vi "mqttTCPIPbrokerConnect.vi"(0 "mqtt in":refnum<class "mqtt.lvclass">, 11 "error in (no error)":errorcluster) -> (4 "mqtt out":refnum<class "mqtt.lvclass">, 15 "error out":errorcluster)   [LabVIEW 2018, in "mqtt.lvclass"]
uses:
  mqtt.lvclass
  mqtt.lvclass/mqtt.ctl
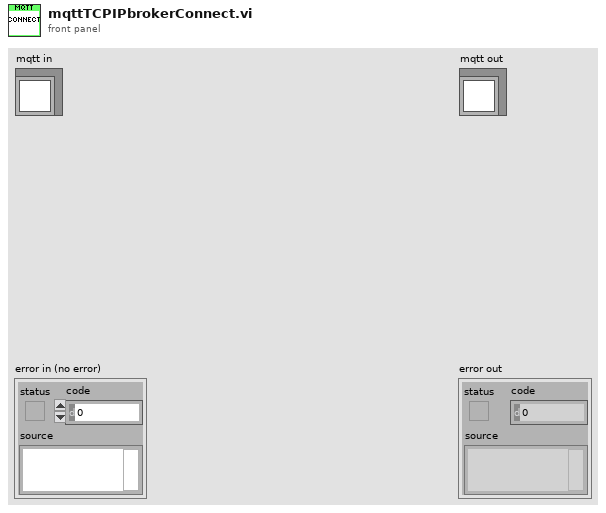
[diagram p1: front panel]
types:
  T1 = typedef "mqttBroker.ctl" = cluster{"address":string, "port":u16, "connTimeout":i32, "writeTimeout":i32, "readTimeout":i32, "subTimeout":i32}
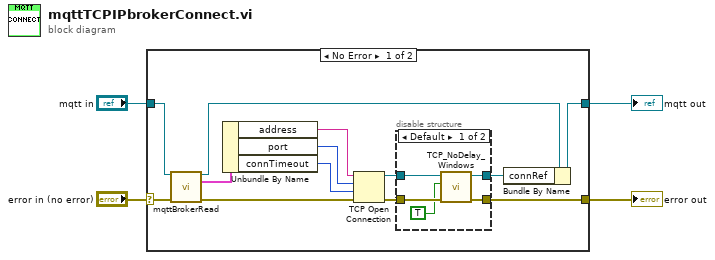
[diagram p0: block diagram]
diagram:
  n1 = case shown="No Error" "error in (no error)" {
    selector: "error in (no error)" -> [w14 w26]
    tunnel: [w15 w26] -> w3
    tunnel: [w5 w25] -> w1
    tunnel: "mqtt in" -> [w9 w25]
    frame No Error {
      n2 = call "mqttBrokerRead.vi"("mqtt in"=w9, "error in (no error)"=w14) -> ("mqtt out"=w7:refnum<class "mqtt.lvclass">, "broker"=w12:T1, "error out"=w13:errorcluster)  [unwired: 11 in]
      n3 = Unbundle By Name(w12) -> ("address"=w11:string, "port"=w10:u16, "connTimeout"=w8:i32)
      n4 = TCP Open Connection(address=w11, remote port or service name=w10, timeout ms (60000)=w8, error in (no error)=w13) -> (connection ID=w17:refnum<k5>, error out=w16:errorcluster)  [unwired: 1 in]
      n5 = disable-structure shown="Default" {
        disable-tunnel: w17 -> [w22 w24]
        disable-tunnel: w16 -> [w21 w23]
        disable-tunnel: [w20 w23] -> w15
        disable-tunnel: [w18 w24] -> w6
        frame condition #0 (active) {
          n6 = call "TCP_NoDelay_Windows.vi"("error in (no error)"=w21, "TCP_NODELAY (true)"=TRUE, "connID"=w22) -> ("error out"=w20:errorcluster, "connID 2"=w18:refnum<k5>)  [unwired: 3 in]
        }
        frame condition #1 {
        }
      }
      n7 = Bundle By Name(cluster=w7, "connRef"=w6) -> (w5:refnum<class "mqtt.lvclass">)
    }
    frame Error {
    }
  }
  "error out" <- w3
  "mqtt out" <- w1
